vi "Empty_queue(SubVI).vi"(8 "error in (no error)":errorcluster, 11 "Queue in":refnum<queue>) -> (3 "Queue out":refnum<queue>)   [LabVIEW 2017]
doc: "SubVI that prevent queue from being closed when not empty"
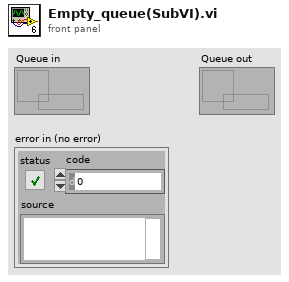
[diagram p1: front panel]
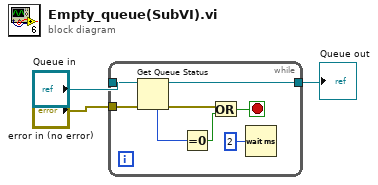
[diagram p0: block diagram]
diagram:
  n1 = while {
    tunnel: "error in (no error)" -> [w9]
    tunnel: "Queue in" -> [w8]
    tunnel: [w7] -> w3
    stop <- w6 stop-if-true
    n2 = Get Queue Status(queue=w8, error in (no error)=w9) -> (queue out=w7:refnum<queue>, error out=w4:errorcluster, # elements in queue=w11:i32)  [unwired: 1 in, 5 out]
    n3 = Equal To 0?(x=w11) -> (x = 0?=w10:bool)
    n4 = Or(x=w4, y=w10) -> (x .or. y?=w6:bool)
    n5 = Wait (ms)(milliseconds to wait=u32 2) -> ()  [unwired: 1 out]
  }
  "Queue out" <- w3
